vi "Configure 4Wire Resistance.vi"(0 "VISA resource name":refnum<visa-resource-name>, 1 "Scan List (Empty)":string, 5 "Enable Offset Compensation (False)":bool, 9 "Dry Circuit Ohms (0: Don't Configure)":u16(ring) items=["Don't Configure", "Enable Dry Circuit Ohms", "Disable Dry Circuit Ohms"], 11 "error in (no error)":errorcluster) -> (4 "VISA resource name out":refnum<visa-resource-name>, 15 "error out":errorcluster)   [LabVIEW 2020, in "Keithley 27XX.lvlib"]
doc: "This VI configures Offset Compensation and Dry Circuit Ohms attributes for 4-Wire Resistance Measurements.\nThe DMM uses the constant-current method to measure resistance from 1 Ohm to 1MOhm. The DMM sources a constant current (I) to the resistance and measures the voltage (V). Resistance (R) is then calculated using the known current and measured voltage (R=V/I). for the 10MOhm and 100MOhm ranges, the ratiometric method is used to measure resistance."
uses:
  <instrlib>/Keithley 27XX/Keithley 27XX.lvlib
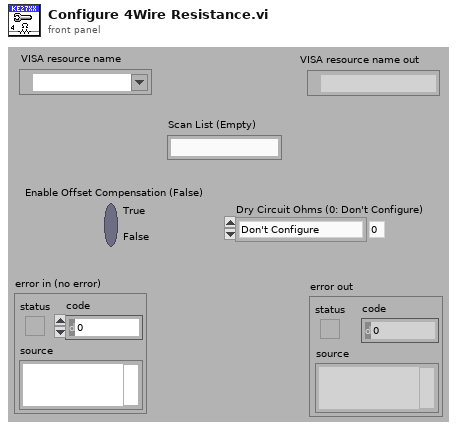
[diagram p1: front panel]
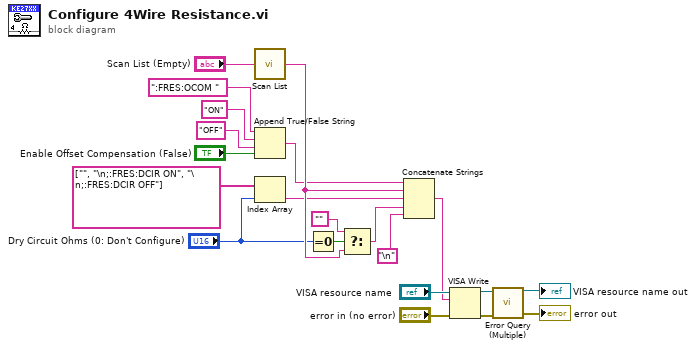
[diagram p0: block diagram]
diagram:
  n1 = call <instrlib>:"Scan List.vi"("Scan List (Empty)"="Scan List (Empty)") -> ("Scan List Out"=w5:string)  [unwired: 14 in]
  n2 = Append True/False String(1:"Enable Offset Compensation (False)", 2:"OFF" ("false string"), 3:"ON" ("true string"), 4:":FRES:OCOM " ("string (\"\")")) -> (0:w2:string)
  n3 = Index Array(array=string[] ["", "\n;:FRES:DCIR ON", "\n;:FRES:DCIR OFF"], index="Dry Circuit Ohms (0: Don't Configure)") -> (element=w3:string)
  n4 = Equal To 0?(x="Dry Circuit Ohms (0: Don't Configure)") -> (x = 0?=w8:bool)
  n5 = Select(t="", s=w8, f=w5) -> (s? t:f=w6:string)
  n6 = Concatenate Strings(w2, w5, w3, w6, "\n") -> (w4:string)
  n7 = VISA Write(VISA resource name="VISA resource name", write buffer=w4, error in (no error)="error in (no error)") -> (VISA resource name out=w14:refnum<visa-resource-name>, error out=w13:errorcluster)  [unwired: 1 out]
  n8 = call <instrlib>:"Error Query (Multiple).vi"("VISA resource name"=w14, "error in (no error)"=w13) -> ("VISA resource name out"=→"VISA resource name out":refnum<visa-resource-name>, "error out"=→"error out":errorcluster)  [unwired: 10 in, 2 out]
